vi "NXTHID-DM.vi"(0 "Input of NXTHID":T1={"Transmit Mode"=1, "Text Data"="NXTHID is typing this...", "Key Modifier"=0, "Keydata"=58} {"Keydata" format="%x"; "Key Modifier" items=["None"=0, "Left Control"=1, "Left Shift"=2, "Left Alt"=4, "Left GUI"=8, "Right Control"=16, "Right Shift"=32, "Right Alt"=64, "Right GUI"=-128]; "Transmit Mode" items=["Direct Keyboard data", "Ascii Text data"]}, 2 "NXT":T3={"Hardware"="NXT", "Flattened String"=""}, 3 "Input Port":T2 items=["Port 1", "Port 2", "Port 3", "Port 4"]) -> (1 "Output of NXTHID":cluster{"Status (boolean)":bool}, 4 "NXT dup":T3={"Hardware"="NXT", "Flattened String"=""})   [LabVIEW 2011]
uses:
  <vilib>/NXT/Subs/LVHSConnector.ctl
  <vilib>/NXT/Block Support/NXT_InputPort.ctl
  <vilib>/NXT/Block Support/HWPage.SensorType.ctl
  <vilib>/NXT/Block Support/HWPage.SensorMode.ctl
panel:
  # "mindsensors.com\nCopyright (c) 2009 by mindsensors.com\nEmail: info (<at>) mindsensors (<dot>) com\n\nThis program is free software. You can redistribute it and/or modify\nit under the terms of the GNU General Public License as published by\nthe Free Software Foundation; version 3 of the License.\nRead the license at: http://www.gnu.org/licenses/gpl.txt"
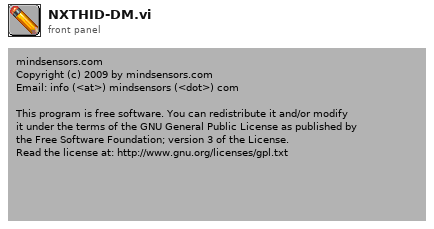
[diagram p1: front panel]
types:
  T1 = cluster{"Transmit Mode":u8, "Text Data":string, "Key Modifier":i8, "Keydata":u8}
  T2 = typedef "NXT_InputPort.ctl" = u8
  T3 = typedef "LVHSConnector.ctl" = cluster{"Hardware":string, "Flattened String":string}
  T4 = typedef "HWPage.SensorType.ctl" = u8
  T5 = typedef "HWPage.SensorMode.ctl" = u8
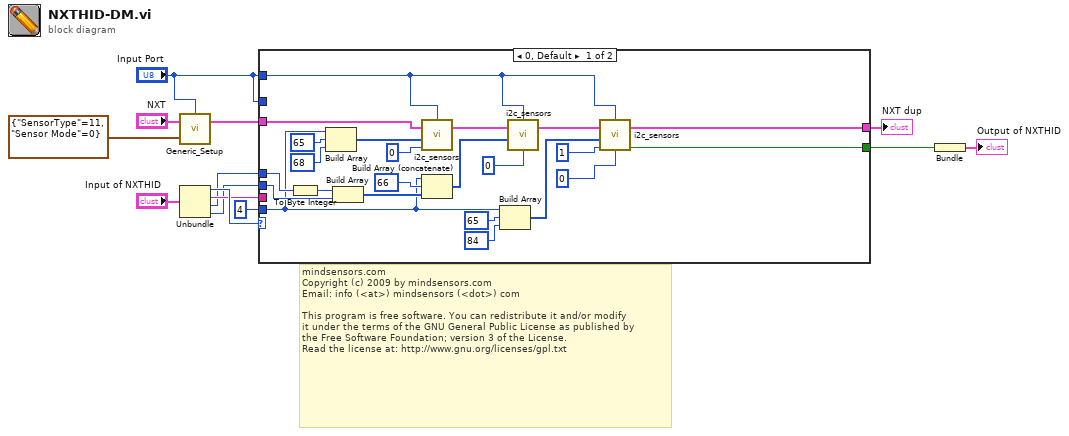
[diagram p0: block diagram]
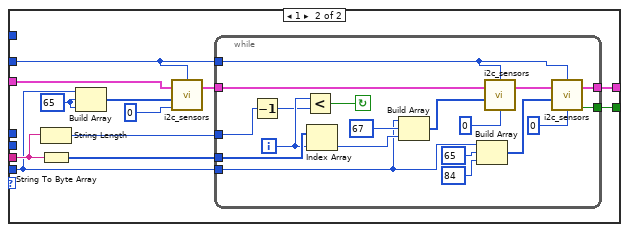
[diagram p2: hidden frame]
diagram:
  # "mindsensors.com\nCopyright (c) 2009 by mindsensors.com\nEmail: info (<at>) mindsensors (<dot>) com\n\nThis program is free software. You can redistribute it and/or modify\nit under the terms of the GNU General Public License as published by\nthe Free Software Foundation; version 3 of the License.\nRead the license at: http://www.gnu.org/licenses/gpl.txt"
  n1 = call <vilib>:"Generic_Setup.vi"("Sensor Setup"=cluster{"SensorType":T4, "Sensor Mode":T5} {"SensorType"=11, "Sensor Mode"=0}, "NXT"="NXT", "Port"="Input Port") -> ("NXT"=w11:T3)  [unwired: 1 out]
  n2 = Unbundle("Input of NXTHID") -> ("Transmit Mode"=w6:u8, "Text Data"=w5:string, "Key Modifier"=w4:i8, "Keydata"=w3:u8)
  n3 = case shown="0, Default" w6 {
    tunnel: 4 -> [w22 w45]
    tunnel: w4 -> [w36 _]
    tunnel: w3 -> [w35 _]
    tunnel: w5 -> [_ w47]
    tunnel: w11 -> [w25 w42]
    tunnel: [w16 w40] -> w9
    tunnel: "Input Port" -> [_ w39]
    tunnel: "Input Port" -> [w19 _]
    tunnel: [w14 w37] -> w2
    frame 0, Default {
      n4 = To Byte Integer(number=w36) -> (8bit integer=w34:i8)
      n5 = Build Array(w22, u8 65 ("register"), u8 68 ("register")) -> (w31:i32[])
      n6 = Build Array(w34, w35) -> (w28:u8[])
      n7 = call <vilib>:"i2c_sensors.vi"("Return Length"=u8 0, "Bytes to Write"=w31, "NXT"=w25, "Port"=w19) -> ("NXT"=w26:T3)  [unwired: 1 in, 2 out]
      n8 = Build Array (concatenate)(w22, u8 66 ("register"), w28) -> (w27:i32[])
      n9 = Build Array(w22, u8 65 ("register"), u8 84 ("register")) -> (w17:i32[])
      n10 = call <vilib>:"i2c_sensors.vi"("Bytes to Write"=w27, "Wait (msec)"=u32 0, "NXT"=w26, "Port"=w19) -> ("NXT"=w18:T3)  [unwired: 1 in, 2 out]
      n11 = call <vilib>:"i2c_sensors.vi"("Return Length"=u8 1, "Bytes to Write"=w17, "Wait (msec)"=u32 0, "NXT"=w18, "Port"=w19) -> ("Success?"=w14:bool, "NXT"=w16:T3)  [unwired: 1 out]
    }
    frame 1 {
      w38 = u8 65 ("register")
      n12 = String Length(string=w47) -> (length=w46:i32)
      n13 = String To Byte Array(string=w47) -> (unsigned byte array=w48:u8[])
      n14 = Build Array(w45, w38, w38) -> (w44:i32[])
      n15 = call <vilib>:"i2c_sensors.vi"("Return Length"=u8 0, "Bytes to Write"=w44, "NXT"=w42, "Port"=w39) -> ("NXT"=w41:T3)  [unwired: 1 in, 2 out]
      n16 = while {
        tunnel: w45 -> [w58]
        tunnel: w48 -> [w66]
        tunnel: w46 -> [w64]
        tunnel: w41 -> [w53]
        tunnel: [w51] -> w40
        tunnel: w39 -> [w50]
        tunnel: [w49] -> w37
        i -> [w63]
        stop <- w62 continue-if-true
        n17 = Decrement(x=w64) -> (x-1=w61:i32)
        n18 = Less?(x=w63, y=w61) -> (x < y?=w62:bool)
        n19 = Index Array(array=w66, index=w63) -> (element=w65:u8)
        n20 = Build Array(w58, u8 67 ("register"), w65) -> (w59:i32[])
        n21 = Build Array(w58, u8 65 ("register"), u8 84 ("register")) -> (w56:i32[])
        n22 = call <vilib>:"i2c_sensors.vi"("Bytes to Write"=w59, "Wait (msec)"=u32 0, "NXT"=w53, "Port"=w50) -> ("NXT"=w52:T3)  [unwired: 1 in, 2 out]
        n23 = call <vilib>:"i2c_sensors.vi"("Bytes to Write"=w56, "Wait (msec)"=u32 0, "NXT"=w52, "Port"=w50) -> ("Success?"=w49:bool, "NXT"=w51:T3)  [unwired: 1 in, 1 out]
      }
    }
  }
  "NXT dup" <- w9
  n24 = Bundle("Success?"=w2) -> (→"Output of NXTHID":cluster{"Success?":bool})  [unwired: 1 in]
